vi "DSF.UDP.Transfer Group.Create.vi"(6 "Cycle Timing Factors":T1={"Decimation"=1, "Offset"=0}, 8 "error in (no error)":errorcluster, 10 "Name":string, 11 "UDP Transfer Configurations":refnum<class "DSF.UDP.Configuration.Transfer.lvclass">[](array[class])) -> (0 "error out":errorcluster, 3 "UDP Transfer Group out":refnum<class "DSF.UDP.Configuration.Transfer Group.lvclass">)   [LabVIEW 2016, in "DSF.UDP.Configuration.Transfer Group.lvclass"]
uses:
  DSF.UDP.Configuration.Transfer Group.lvclass
  C:/Git/SourceTree/DSF/Source/Shared/Classes/Transfer Group/DSF.Shared.Configuration.Transfer Group.lvclass
  DSF.UDP.Configuration.Transfer.lvclass
  C:/Git/SourceTree/DSF/Source/Shared/Classes/Transfer/DSF.Shared.Configuration.Transfer.lvclass
  Source/Shared/Typedefs/DSF.Shared.Typedefs.Cycle Timing Factors.ctl
  Source/Shared/Classes/Transfer Group/DSF.Shared.Configuration.Transfer Group.lvclass
  Source/DSF.Shared.lvlib
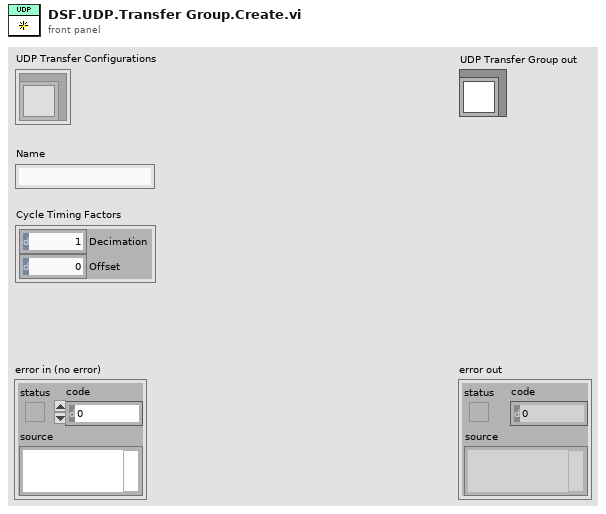
[diagram p1: front panel]
types:
  T1 = typedef "DSF.Shared.lvlib/DSF.Shared.Typedefs.Cycle Timing Factors.ctl" = cluster{"Decimation":u64, "Offset":u64}
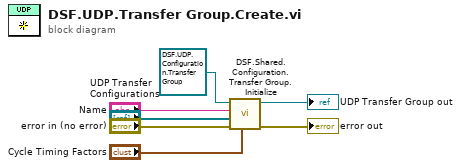
[diagram p0: block diagram]
diagram:
  n1 = call "DSF.Shared.Configuration.Transfer Group.Initialize.vi"("Cycle Timing Factors"="Cycle Timing Factors", "error in (no error)"="error in (no error)", "Transfer Configurations"="UDP Transfer Configurations", "Name"="Name", "Transfer Group Configuration in"=refnum<class "DSF.UDP.Configuration.Transfer Group.lvclass"> refnum ("UDP Transfer Group in")) -> ("error out"=→"error out":errorcluster, "Transfer Group Configuration out"=→"UDP Transfer Group out":refnum<class "DSF.UDP.Configuration.Transfer Group.lvclass">)  [unwired: 5 in]
